vi "NEO Get Sensor Values.vi"(11 "Swerve Motors":T1={"Drive Motors (NEO)"={"Left Front"={"DeviceStatus"={"status"=FALSE, "code"=0, "source"=""}, "Type"=enum."PWM", "PWM"={"PWM Channel"=enum."Invalid", "DeadBand"={"Name"="", "maxPositivePwm"=0, "minPositivePwm"=0, "centerPwm"=0, "maxNegativePwm"=0, "minNegativePwm"=0, "angularRange"=0}}, "CAN"={"Device Number"=0, "SetOutput VI Ref"=variant, "GetOutput VI Ref"=variant, "Enable VI Ref"=variant, "Disable VI Ref"=variant, "Data"=variant}, "Invert"=FALSE, "DIO PWM"={"PWM \"Enable\" Channel"=enum."Invalid", "DIOChannel"=enum."Invalid", "PWM Rate"=0.0}}, "Left Back"={"DeviceStatus"={"status"=FALSE, "code"=0, "source"=""}, "Type"=enum."PWM", "PWM"={"PWM Channel"=enum."Invalid", "DeadBand"={"Name"="", "maxPositivePwm"=0, "minPositivePwm"=0, "centerPwm"=0, "maxNegativePwm"=0, "minNegativePwm"=0, "angularRange"=0}}, "CAN"={"Device Number"=0, "SetOutput VI Ref"=variant, "GetOutput VI Ref"=variant, "Enable VI Ref"=variant, "Disable VI Ref"=variant, "Data"=variant}, "Invert"=FALSE, "DIO PWM"={"PWM \"Enable\" Channel"=enum."Invalid", "DIOChannel"=enum."Invalid", "PWM Rate"=0.0}}, "Right Front"={"DeviceStatus"={"status"=FALSE, "code"=0, "source"=""}, "Type"=enum."PWM", "PWM"={"PWM Channel"=enum."Invalid", "DeadBand"={"Name"="", "maxPositivePwm"=0, "minPositivePwm"=0, "centerPwm"=0, "maxNegativePwm"=0, "minNegativePwm"=0, "angularRange"=0}}, "CAN"={"Device Number"=0, "SetOutput VI Ref"=variant, "GetOutput VI Ref"=variant, "Enable VI Ref"=variant, "Disable VI Ref"=variant, "Data"=variant}, "Invert"=FALSE, "DIO PWM"={"PWM \"Enable\" Channel"=enum."Invalid", "DIOChannel"=enum."Invalid", "PWM Rate"=0.0}}, "Right Back"={"DeviceStatus"={"status"=FALSE, "code"=0, "source"=""}, "Type"=enum."PWM", "PWM"={"PWM Channel"=enum."Invalid", "DeadBand"={"Name"="", "maxPositivePwm"=0, "minPositivePwm"=0, "centerPwm"=0, "maxNegativePwm"=0, "minNegativePwm"=0, "angularRange"=0}}, "CAN"={"Device Number"=0, "SetOutput VI Ref"=variant, "GetOutput VI Ref"=variant, "Enable VI Ref"=variant, "Disable VI Ref"=variant, "Data"=variant}, "Invert"=FALSE, "DIO PWM"={"PWM \"Enable\" Channel"=enum."Invalid", "DIOChannel"=enum."Invalid", "PWM Rate"=0.0}}}, "Steer Motors (NEO)"={"Left Front"={"DeviceStatus"={"status"=FALSE, "code"=0, "source"=""}, "Type"=enum."PWM", "PWM"={"PWM Channel"=enum."Invalid", "DeadBand"={"Name"="", "maxPositivePwm"=0, "minPositivePwm"=0, "centerPwm"=0, "maxNegativePwm"=0, "minNegativePwm"=0, "angularRange"=0}}, "CAN"={"Device Number"=0, "SetOutput VI Ref"=variant, "GetOutput VI Ref"=variant, "Enable VI Ref"=variant, "Disable VI Ref"=variant, "Data"=variant}, "Invert"=FALSE, "DIO PWM"={"PWM \"Enable\" Channel"=enum."Invalid", "DIOChannel"=enum."Invalid", "PWM Rate"=0.0}}, "Left Back"={"DeviceStatus"={"status"=FALSE, "code"=0, "source"=""}, "Type"=enum."PWM", "PWM"={"PWM Channel"=enum."Invalid", "DeadBand"={"Name"="", "maxPositivePwm"=0, "minPositivePwm"=0, "centerPwm"=0, "maxNegativePwm"=0, "minNegativePwm"=0, "angularRange"=0}}, "CAN"={"Device Number"=0, "SetOutput VI Ref"=variant, "GetOutput VI Ref"=variant, "Enable VI Ref"=variant, "Disable VI Ref"=variant, "Data"=variant}, "Invert"=FALSE, "DIO PWM"={"PWM \"Enable\" Channel"=enum."Invalid", "DIOChannel"=enum."Invalid", "PWM Rate"=0.0}}, "Right Front"={"DeviceStatus"={"status"=FALSE, "code"=0, "source"=""}, "Type"=enum."PWM", "PWM"={"PWM Channel"=enum."Invalid", "DeadBand"={"Name"="", "maxPositivePwm"=0, "minPositivePwm"=0, "centerPwm"=0, "maxNegativePwm"=0, "minNegativePwm"=0, "angularRange"=0}}, "CAN"={"Device Number"=0, "SetOutput VI Ref"=variant, "GetOutput VI Ref"=variant, "Enable VI Ref"=variant, "Disable VI Ref"=variant, "Data"=variant}, "Invert"=FALSE, "DIO PWM"={"PWM \"Enable\" Channel"=enum."Invalid", "DIOChannel"=enum."Invalid", "PWM Rate"=0.0}}, "Right Back"={"DeviceStatus"={"status"=FALSE, "code"=0, "source"=""}, "Type"=enum."PWM", "PWM"={"PWM Channel"=enum."Invalid", "DeadBand"={"Name"="", "maxPositivePwm"=0, "minPositivePwm"=0, "centerPwm"=0, "maxNegativePwm"=0, "minNegativePwm"=0, "angularRange"=0}}, "CAN"={"Device Number"=0, "SetOutput VI Ref"=variant, "GetOutput VI Ref"=variant, "Enable VI Ref"=variant, "Disable VI Ref"=variant, "Data"=variant}, "Invert"=FALSE, "DIO PWM"={"PWM \"Enable\" Channel"=enum."Invalid", "DIOChannel"=enum."Invalid", "PWM Rate"=0.0}}}, "Pigeon2"={"CANbus Name"="", "Device Encoding"=0, "Device Name"=""}, "Radii (ft)"={"Left Front Position"=[], "Left Back Position"=[], "Right Front Position"=[], "Right Back Position"=[]}} {"Radii (ft)"."Right Back Position" format="%.2f"; "Radii (ft)"."Right Front Position" format="%.2f"; "Radii (ft)"."Left Back Position" format="%.2f"; "Radii (ft)"."Left Front Position" format="%.2f"}) -> (2 "Steer Angles (degrees)":T10, 3 "Drive Velocities (ft/s)":T10)   [LabVIEW 2025]
uses:
  Type Definitions/Hardware/Swerve Drives/(NEO-NEO-ThroughBore-Pigeon2) Swerve.ctl
  Type Definitions/Hardware/4 Motor Sets/(NEO & NEO 550) 4 Motor Set.ctl
  <vilib>/Rock Robotics/WPI/MotorControl/WPI_MotorControlDeviceRef.ctl
  <vilib>/Rock Robotics/WPI/MotorControl/WPI_MotorControlType.ctl
  <vilib>/Rock Robotics/SystemInterfaces/DIO/FPGA_DIOPWMChannel.ctl
  <vilib>/Rock Robotics/WPI/PWM/WPI_PWMDeadband.ctl
  <vilib>/Rock Robotics/SystemInterfaces/DIO/FPGA_DIOChannel.ctl
  <vilib>/Rock Robotics/WPI/ThirdParty/Phoenix6/DeviceReference.ctl
  Type Definitions/Data/Pod Positions.ctl
  <vilib>/Rock Robotics/WPI/ThirdParty/REV Robotics/REVLib/SubVI/Public/SPARK Get Encoder Status Velocity.vi
  <vilib>/Rock Robotics/WPI/ThirdParty/REV Robotics/REVLib/SubVI/Public/SPARK Get Encoder Status Position.vi
panel:
  in  "Max Delay":u32
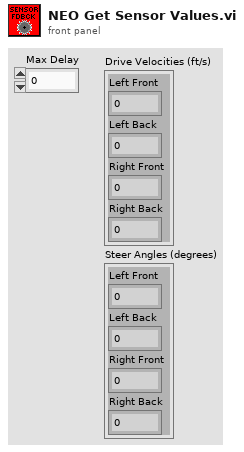
[diagram p1: front panel]
types:
  T1 = typedef "(NEO-NEO-ThroughBore-Pigeon2) Swerve.ctl" = cluster{"Drive Motors (NEO)":T2, "Steer Motors (NEO)":T2, "Pigeon2":T8, "Radii (ft)":T9}
  T2 = typedef "(NEO & NEO 550) 4 Motor Set.ctl" = cluster{"Left Front":T3, "Left Back":T3, "Right Front":T3, "Right Back":T3}
  T3 = typedef "WPI_MotorControlDeviceRef.ctl" = cluster{"DeviceStatus":errorcluster, "Type":T4, "PWM":cluster{"PWM Channel":T5, "DeadBand":T6}, "CAN":cluster{"Device Number":u8, "SetOutput VI Ref":variant, "GetOutput VI Ref":variant, "Enable VI Ref":variant, "Disable VI Ref":variant, "Data":variant}, "Invert":bool, "DIO PWM":cluster{"PWM \"Enable\" Channel":T5, "DIOChannel":T7, "PWM Rate":dbl}}
  T4 = typedef "WPI_MotorControlType.ctl" = enum16{"PWM", "CAN", "DIO PWM"}
  T5 = typedef "FPGA_DIOPWMChannel.ctl" = enum8{"PWM 0", "PWM 1", "PWM 2", "PWM 3", "PWM 4", "PWM 5", "PWM 6", "PWM 7", "PWM 8", "PWM 9", "PWM MXP 0", "PWM MXP 1", "PWM MXP 2", "PWM MXP 3", "PWM MXP 4", "PWM MXP 5", "PWM MXP 6", "PWM MXP 7", "PWM MXP 8", "PWM MXP 9", "Invalid"}
  T6 = typedef "WPI_PWMDeadband.ctl" = cluster{"Name":string, "maxPositivePwm":i32, "minPositivePwm":i32, "centerPwm":i32, "maxNegativePwm":i32, "minNegativePwm":i32, "angularRange":u16}
  T7 = typedef "FPGA_DIOChannel.ctl" = enum8{"DIO 0", "DIO 1", "DIO 2", "DIO 3", "DIO 4", "DIO 5", "DIO 6", "DIO 7", "DIO 8", "DIO 9", "DIO MXP 0", "DIO MXP 1", "DIO MXP 2", "DIO MXP 3", "DIO MXP 4", "DIO MXP 5", "DIO MXP 6", "DIO MXP 7", "DIO MXP 8", "DIO MXP 9", "DIO MXP 10", "DIO MXP 11", "DIO MXP 12", "DIO MXP 13", "DIO MXP 14", "DIO MXP 15", "SPI Port CS1", "SPI Port CS2", "SPI Port CS3", "SPI Port MISO", "SPI Port MOSI", "Invalid"}
  T8 = typedef "DeviceReference.ctl" = cluster{"CANbus Name":string, "Device Encoding":u32, "Device Name":string}
  T9 = typedef "Pod Positions.ctl" = cluster{"Left Front Position":dbl[], "Left Back Position":dbl[], "Right Front Position":dbl[], "Right Back Position":dbl[]}
  T10 = cluster{"Left Front":dbl, "Left Back":dbl, "Right Front":dbl, "Right Back":dbl}
  T11 = cluster{"[0]":dbl, "[1]":dbl, "[2]":dbl, "[3]":dbl}
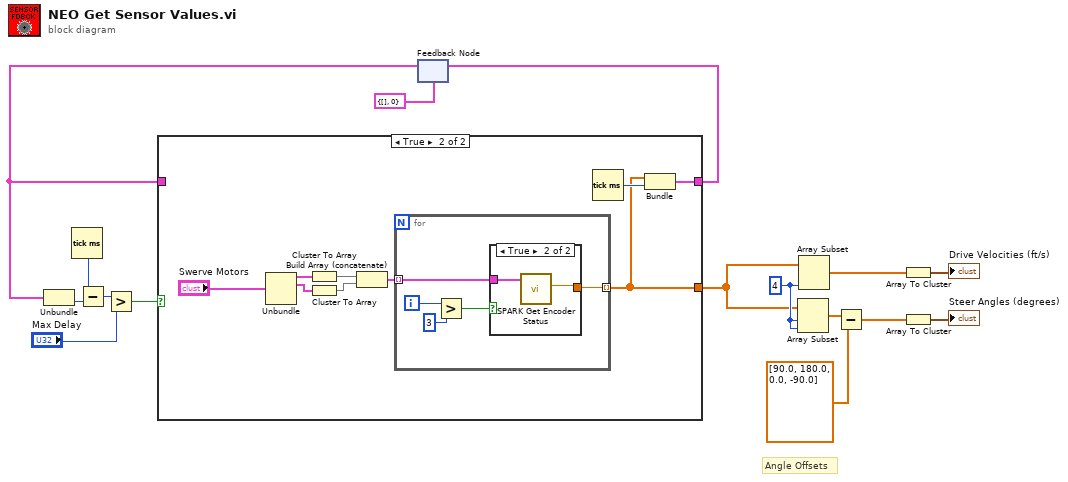
[diagram p0: block diagram]
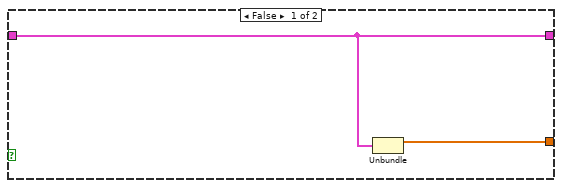
[diagram p2: hidden frame]
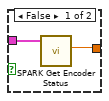
[diagram p3: hidden frame]
diagram:
  w15 = 4 ("length")
  # "Angle Offsets"
  n1 = Tick Count (ms)() -> (millisecond timer value=w7:u32)
  n2 = feedback #1(cluster{dbl[], "millisecond timer value":u32} {[], "millisecond timer value"=0}) -> (w6:cluster{dbl[], "millisecond timer value":u32})
  n3 = Unbundle(w6) -> ("millisecond timer value"=w5:u32)  [unwired: 1 out]
  n4 = Subtract(x=w7, y=w5) -> (x-y=w4:u32)
  n5 = Greater?(x=w4, y="Max Delay") -> (0:w2:bool)
  n6 = case shown="True" w2 {
    tunnel: [w17 w20] -> w9
    tunnel: [w18 w19] -> w8
    tunnel: w6 -> [w18 _]
    frame False {
      n7 = Unbundle(w18) -> (w17:dbl[])  [unwired: 1 out]
    }
    frame True {
      n8 = Unbundle("Swerve Motors") -> ("Drive Motors (NEO)"=w27:T2, "Steer Motors (NEO)"=w26:T2)  [unwired: 2 out]
      n9 = Cluster To Array(cluster=w27) -> (array=w25:T3[])
      n10 = Cluster To Array(cluster=w26) -> (array=w24:T3[])
      n11 = Build Array (concatenate)(w25, w24) -> (w23:T3[])
      n12 = for {
        tunnel: w23 -> [w29] mode=indexing
        tunnel: [w28] -> w20 mode=indexing
        i -> [w31]
        n13 = Greater?(x=w31, y=3) -> (0:w30:bool)
        n14 = case shown="True" w30 {
          tunnel: w29 -> [w34 w36]
          tunnel: [w33 w35] -> w28
          frame False {
            n15 = call-poly <vilib>:"SPARK Get Encoder Status.vi"("MotorControlDevRef in"=w34) -> ("Sensor Velocity"=w33:dbl)  [unwired: 7 in, 3 out]
          }
          frame True {
            n16 = call-poly <vilib>:"SPARK Get Encoder Status.vi"("MotorControlDevRef in"=w36) -> ("Sensor Position"=w35:dbl)  [unwired: 7 in, 3 out]
          }
        }
      }
      n17 = Tick Count (ms)() -> (millisecond timer value=w21:u32)
      n18 = Bundle(w20, "millisecond timer value"=w21) -> (w19:cluster{dbl[], "millisecond timer value":u32})  [unwired: 1 in]
    }
  }
  n19 = feedback-in #1(w8) -> ()
  n20 = Array Subset(array=w9, index=w15, length=w15) -> (w12:dbl[])
  n21 = Array Subset(array=w9, length=w15) -> (w16:dbl[])  [unwired: 1 in]
  n22 = Subtract(x=w12, y=dbl[] [90.0, 180.0, 0.0, -90.0]) -> (x-y=w10:dbl[])
  n23 = Array To Cluster(array=w16) -> (cluster=→"Drive Velocities (ft/s)":T11)
  n24 = Array To Cluster(array=w10) -> (cluster=→"Steer Angles (degrees)":T11)
